vi "Espresso.vi"(8 "error in (no error)":errorcluster caption="错误输入（无错误）", 11 "Espresso 输入":refnum<class "Espresso.lvclass">) -> (0 "error out":errorcluster caption="错误输出", 3 "Espresso 输出":refnum<class "Espresso.lvclass">)   [LabVIEW 2016, in "Espresso.lvclass"]
uses:
  Espresso.lvclass
  Beverage.lvclass/Beverage.ctl
  Beverage.lvclass
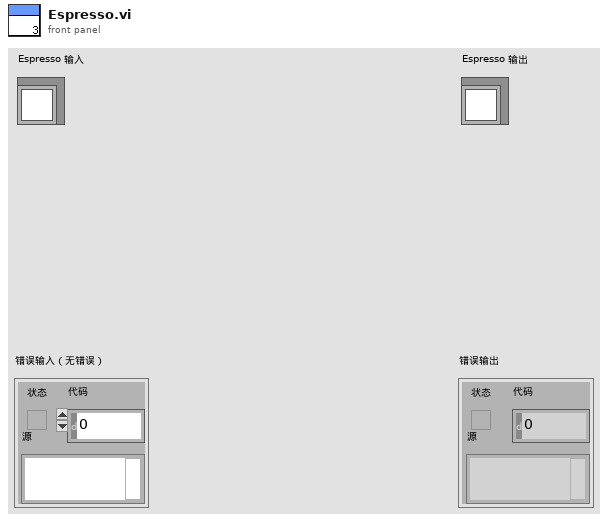
[diagram p1: front panel]
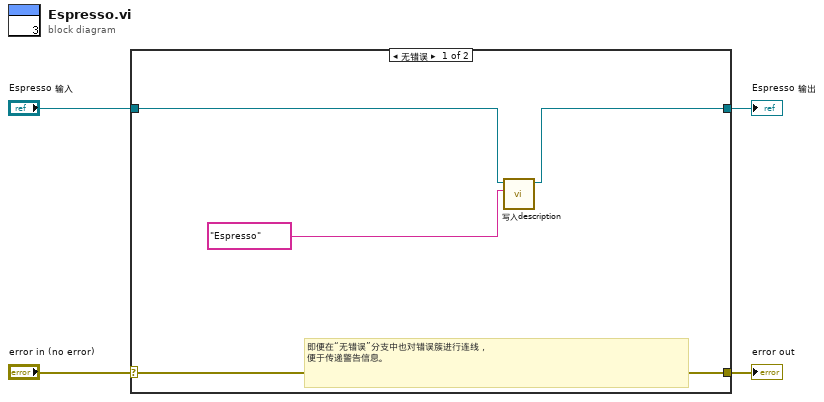
[diagram p0: block diagram]
diagram:
  n1 = case shown="无错误" "error in (no error)" {
    selector: "error in (no error)" -> [w8 w10]
    tunnel: [w8 w10] -> w3
    tunnel: [w5 w9] -> w1
    tunnel: "Espresso 输入" -> [w6 w9]
    frame No Error {
      # "即便在“无错误”分支中也对错误簇进行连线，\n便于传递警告信息。"
      n2 = call "写入description.vi"("description"="Espresso" ("Description"), "Beverage输入"=w6) -> ("Beverage输出"=w5:refnum<class "Espresso.lvclass">)  [unwired: 8 in, 1 out]
    }
    frame Error {
    }
  }
  "error out" <- w3
  "Espresso 输出" <- w1
